vi "execution class name.vi"(8 "error in":errorcluster, 11 "Custom Controller Module configuration in":refnum<class "Custom Controller Module configuration.lvclass">) -> (0 "error out":errorcluster, 2 "class name":string, 3 "Custom Controller Module configuration out":refnum<class "Custom Controller Module configuration.lvclass">)   [LabVIEW 2013, in "Custom Controller Module configuration.lvclass"]
doc: "Provides an interface for determining the module runtime class associated with this module configuration. This class name can then be used to dynamically load or locate the runtime class for initialization purposes."
uses:
  Custom Controller Module configuration.lvclass
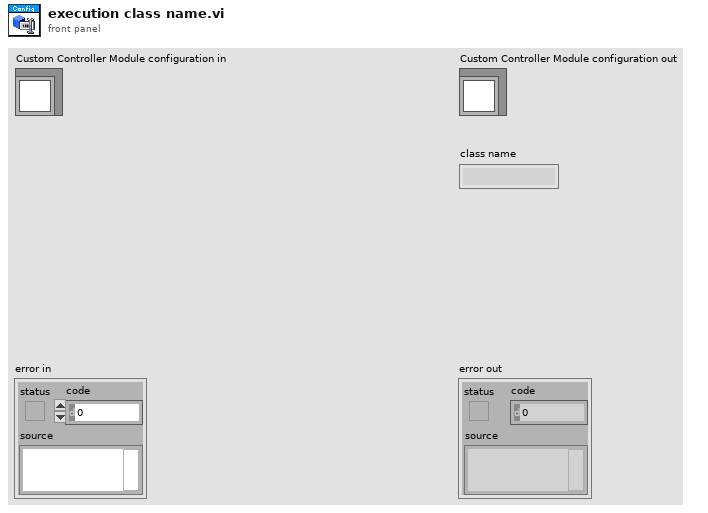
[diagram p1: front panel]
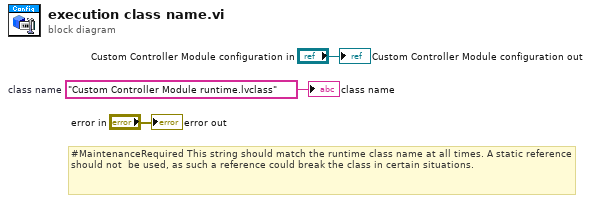
[diagram p0: block diagram]
diagram:
  w1 = "Custom Controller Module runtime.lvclass"  # class name
  # "#MaintenanceRequired This string should match the runtime class name at all times. A static reference should not  be used, as such a reference could break the class in certain situations."
  "error out" <- "error in"
  "Custom Controller Module configuration out" <- "Custom Controller Module configuration in"
  "class name" <- w1
